vi "DataLogger.constructor.vi"(0 "name":string, 2 "data in":string, 5 "error in (no error)":errorcluster) -> (14 "i ref out":refnum<vi>, 16 "data out":string, 19 "error out":errorcluster)   [LabVIEW 2014, in "DataLogger.lvlib"]
doc: "This is the constructor of a class.\n\nLicense Agreement for this software:\n\nCopyright (C)\nGesellschaft für Schwerionenforschung, GSI\nPlanckstr. 1\n64291 Darmstadt\nGermany\n\nContact: D.Beck@gsi.de \n\nThis program is free software; you can redistribute it and/or modify it under the terms of the \nGNU General Public License as published by the Free Software Foundation; either version 2 of \nthe license, or (at your option) any later version.\n\nThis program is distributed in the hope that it will be useful, but WITHOUT ANY WARRANTY; \nwithout even the implied warranty of MERCHANTABILITY or FITNESS FOR A PARTICULAR PURPOSE. See the GNU General License for more details (http://www.gnu.org).\n\nGesellschaft für Schwerionenforschung, GSI\nPlanckstr. 1, 64291 Darmstadt, Germany\nFor all questions and ideas contact: M.Richter@gsi.de, H.Brand@gsi.de or D.Beck@gsi.de.\nLast update: 16-JUN-2004"
uses:
  DataLogger.lvlib
  CS_Core/CSApplicationBaseClasses/DeviceBase/DeviceBase.myEventNames.ctl
  CS_Core/CSApplicationBaseClasses/DeviceBase/DeviceBase.lvlib
  CS_Core/CSSystem/CSSystemLib/CSSystemLib.lvlib
  CSlibraries-extern/DimLVEvent/LVDimInterface/LVDimInterface.lvlib
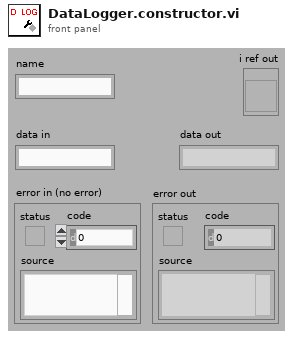
[diagram p1: front panel]
types:
  T1 = enum16{"SetAttribute", "GetAttribute", "CreateAttribute", "DestroyAttribute", "DestroyAllAtributes"}
  T2 = typedef "DeviceBase.lvlib/DeviceBase.myEventNames.ctl" = enum16{"lvmsg://Initialize", "lvmsg://Close", "lvmsg://Configure", "lvmsg://Reset", "lvmsg://IDQuery"}
  T3 = typedef "DataLogger.lvlib/DataLogger.i attribute.ctl" = cluster{"Service Names":string[], "Path":string[], "Service Alarm Index":i32[], "Service Alarm Limit1":dbl[], "Service Alarm Limit2":dbl[], "Service Alarm Indicator":bool[], "alarmID":i32, "pathID":i32, "SoundDeviceID":i32, "SoundFile":string, "SoundID":i32, "SoundFileID":i32}
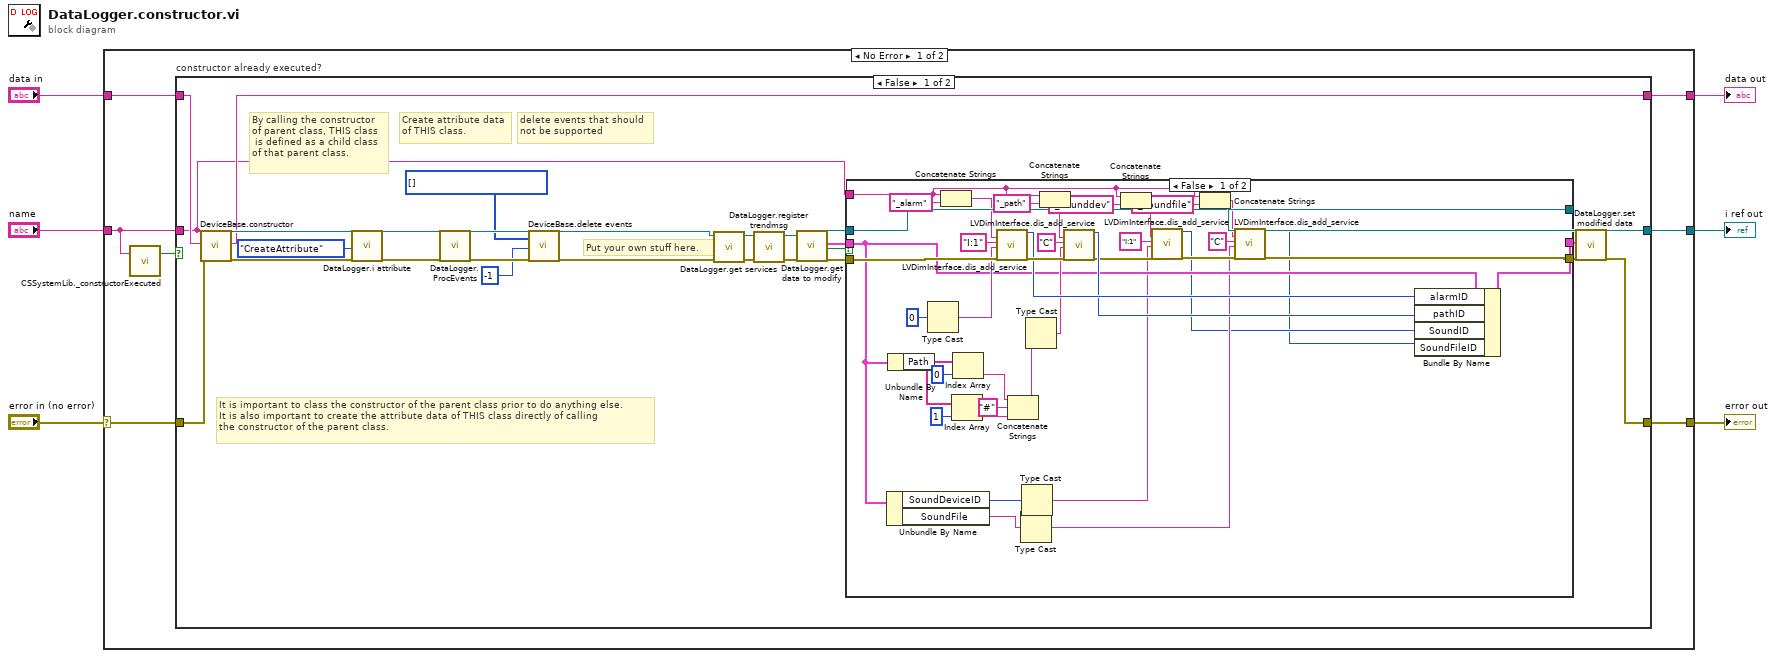
[diagram p0: block diagram]
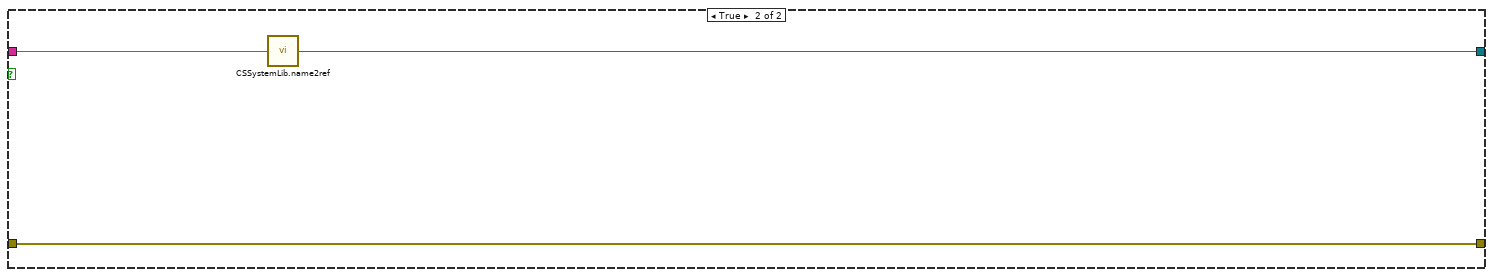
[diagram p3: hidden frame]
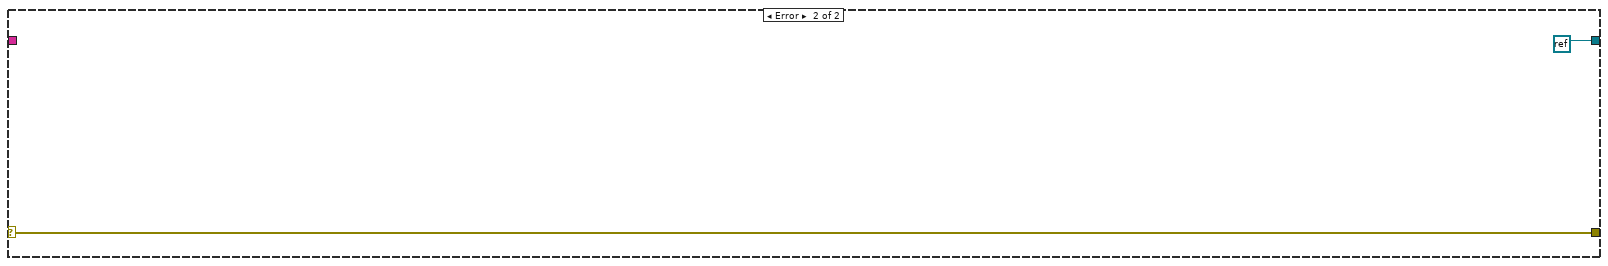
[diagram p4: hidden frame]
diagram:
  n1 = case shown="No Error" "error in (no error)" {
    selector: "error in (no error)" -> [w11 w87]
    tunnel: "name" -> [w10 _]
    tunnel: [w13 refnum<k0> refnum ("Not a Refnum Constant")] -> w5
    tunnel: [w12 w87] -> w4
    tunnel: "data in" -> [w8 _]
    tunnel: [w7 _] -> w1
    frame No Error {
      n2 = call "CSSystemLib._constructorExecuted.vi"("name"=w10) -> ("constructor executed?"=w9:bool)  [unwired: 18 in]
      n3 = case "constructor already executed?" shown="False" w9 {
        tunnel: w10 -> [w15 w86]
        tunnel: [w18 w85] -> w13
        tunnel: [w19 w84] -> w12
        tunnel: w11 -> [w36 w84]
        tunnel: w8 -> [w35 _]
        tunnel: [w30 _] -> w7
        frame False {
          w32 = T2[] [] items=["lvmsg://Initialize", "lvmsg://Close", "lvmsg://Configure", "lvmsg://Reset", "lvmsg://IDQuery"] ("events")
          # "delete events that should\nnot be supported"
          # "It is important to class the constructor of the parent class prior to do anything else.\nIt is also important to create the attribute data of THIS class directly of calling\nthe constructor of the parent class."
          # "Put your own stuff here."
          # "Create attribute data\nof THIS class."
          # "By calling the constructor\nof parent class, THIS class\n is defined as a child class\nof that parent class."
          n4 = call "DeviceBase.constructor.vi"("name"=w15, "data in"=w35, "error in (no error)"=w36) -> ("i ref out"=w41:refnum<vi>, "data out"=w30:string, "error out"=w40:errorcluster)  [unwired: 14 in]
          n5 = call "DataLogger.i attribute.vi"("VI Refnum"=w41, "Action"=T1."CreateAttribute", "error in (no error)"=w40) -> ("VI Refnum out"=w38:refnum<vi>, "error out"=w37:errorcluster)  [unwired: 14 in, 1 out]
          n6 = call "DataLogger.ProcEvents.vi"("i ref in"=w38, "error in (no error)"=w37) -> ("i ref out"=w34:refnum<vi>, "error out"=w33:errorcluster)  [unwired: 16 in]
          n7 = call "DeviceBase.delete events.vi"("i ref in"=w34, "events"=w32, "ms timeout (10000)"=-1, "error in (no error)"=w33) -> ("i ref out"=w29:refnum<vi>, "error out"=w28:errorcluster)  [unwired: 13 in, 1 out]
          n8 = call "DataLogger.get services.vi"("error in (no error)"=w28, "i ref in"=w29) -> ("error out"=w26:errorcluster, "i ref out"=w27:refnum<vi>)  [unwired: 8 in]
          n9 = call "DataLogger.register trendmsg.vi"("error in (no error)"=w26, "i ref in"=w27) -> ("error out"=w24:errorcluster, "i ref out"=w25:refnum<vi>)  [unwired: 8 in]
          n10 = call "DataLogger.get data to modify.vi"("i ref in"=w25, "error in (no error)"=w24) -> ("i ref out"=w21:refnum<vi>, "i attribute"=w16:T3, "timed out"=w22:bool, "error out"=w23:errorcluster)  [unwired: 14 in]
          n11 = case shown="False" w22 {
            tunnel: [w56 w82] -> w20
            tunnel: w15 -> [w52 _]
            tunnel: w23 -> [w79 w82]
            tunnel: w21 -> [w78 w83]
            tunnel: [w78 w83] -> w17
            tunnel: w16 -> [w49 w81]
            tunnel: [w65 w81] -> w14
            frame False {
              n12 = Unbundle By Name(w49) -> ("SoundDeviceID"=w48:i32, "SoundFile"=w46:string)
              n13 = Unbundle By Name(w49) -> ("Path"=w64:string[])
              n14 = Type Cast(x=0) -> (*(type *) &x=w69:string)  [unwired: 1 in]
              n15 = Concatenate Strings(w52, "_alarm" ("string")) -> (w76:string)
              n16 = Index Array(array=w64, index=1) -> (element=w60:string)
              n17 = Index Array(array=w64, index=0 ("length")) -> (element=w62:string)
              n18 = call "LVDimInterface.dis_add_service.vi"("serviceName"=w76, "typeDescriptor"="I:1", "data"=w69, "error in (no error)"=w79) -> ("my_serviceID"=w71:i32, "error out"=w77:errorcluster)  [unwired: 14 in]
              n19 = Concatenate Strings(w62, "#" ("string"), w60) -> (w61:string)
              n20 = Type Cast(x=w46) -> (*(type *) &x=w45:string)  [unwired: 1 in]
              n21 = Type Cast(x=w48) -> (*(type *) &x=w47:string)  [unwired: 1 in]
              n22 = Type Cast(x=w61) -> (*(type *) &x=w67:string)  [unwired: 1 in]
              n23 = Concatenate Strings(w52, "_path" ("string")) -> (w74:string)
              n24 = call "LVDimInterface.dis_add_service.vi"("serviceName"=w74, "typeDescriptor"="C", "data"=w67, "error in (no error)"=w77) -> ("my_serviceID"=w70:i32, "error out"=w58:errorcluster)  [unwired: 14 in]
              n25 = Concatenate Strings(w52, "_sounddev" ("string")) -> (w55:string)
              n26 = call "LVDimInterface.dis_add_service.vi"("serviceName"=w55, "typeDescriptor"="I:1", "data"=w47, "error in (no error)"=w58) -> ("my_serviceID"=w43:i32, "error out"=w57:errorcluster)  [unwired: 14 in]
              n27 = Concatenate Strings(w52, "_soundfile" ("string")) -> (w53:string)
              n28 = call "LVDimInterface.dis_add_service.vi"("serviceName"=w53, "typeDescriptor"="C", "data"=w45, "error in (no error)"=w57) -> ("my_serviceID"=w42:i32, "error out"=w56:errorcluster)  [unwired: 14 in]
              n29 = Bundle By Name(cluster=w49, "alarmID"=w71, "pathID"=w70, "SoundID"=w43, "SoundFileID"=w42) -> (w65:T3)
            }
            frame True {
            }
          }
          n30 = call "DataLogger.set modified data.vi"("i ref in"=w17, "i attribute"=w14, "error in (no error)"=w20) -> ("i ref out"=w18:refnum<vi>, "error out"=w19:errorcluster)  [unwired: 15 in]
        }
        frame True {
          n31 = call "CSSystemLib.name2ref.vi"("name"=w86) -> ("obj refnum"=w85:refnum<vi>)
        }
      }
    }
    frame Error {
    }
  }
  "i ref out" <- w5
  "error out" <- w4
  "data out" <- w1
